vi "Remove Start&End.vi"(11 "Lumps List":string[](array[string])) -> (3 "filtered array":string[](array[string]))   [LabVIEW 2017]
uses:
  <userlib>/_OpenG.lib/array/array.llb/Filter 1D Array (String)__ogtk.vi
  <vilib>/regexp/Match Regular Expression.xnode
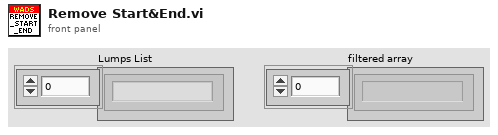
[diagram p1: front panel]
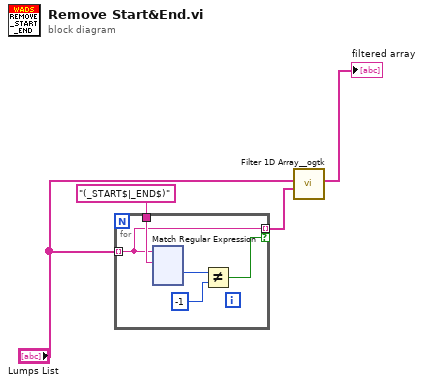
[diagram p0: block diagram]
diagram:
  n1 = for {
    tunnel: "Lumps List" -> [w6] mode=indexing
    tunnel: "(_START$|_END$)" ("format string") -> [w7]
    tunnel: [w6] -> w1 mode=indexing if=w5
    n2 = xnode "Match Regular Expression"("input string"=w6, "regular expression"=w7) -> ("offset past match"=w9:i32)  [unwired: 4 in, 4 out]
    n3 = Not Equal?(x=w9, y=-1) -> (x != y?=w5:bool)
  }
  n4 = call-poly <userlib>:"Filter 1D Array__ogtk.vi"("items to filter"=w1, "array"="Lumps List") -> ("filtered array"=→"filtered array":string[])  [unwired: 4 in, 1 out]
